vi "KB- 颜色分类.vi"(10 "Fitted Circle (Inner Find Circular Edge 2)":T3, 11 "image in":T1(plugin-control)) -> (2 "输出簇":cluster{"金色个数":i32, "银色个数":i32, "黑色个数":i32}, 3 "image in 2":T1(plugin-control))   [LabVIEW 2015]
uses:
  <vilib>/vision/NI_Vision_Development_Module.lvlib
panel:
  out "黑色":i32
  out "银色":i32
  out "金色个数":i32
  out "数组":T2(array[cluster])
  out "Image Pixels (U32)":u32[][](array[numeric])
  # "Overview: Demonstrates how to use the IMAQ Classify function with a color classifier file to classify the color within a Region of Interest (ROI).\nRequirements: Vision Development Software.\nInstructions:\n1. Run the VI.\n2. Draw a ROI in the image to see what class the color is associated with and the score. Hold down <Ctrl> to select more than one ROI."
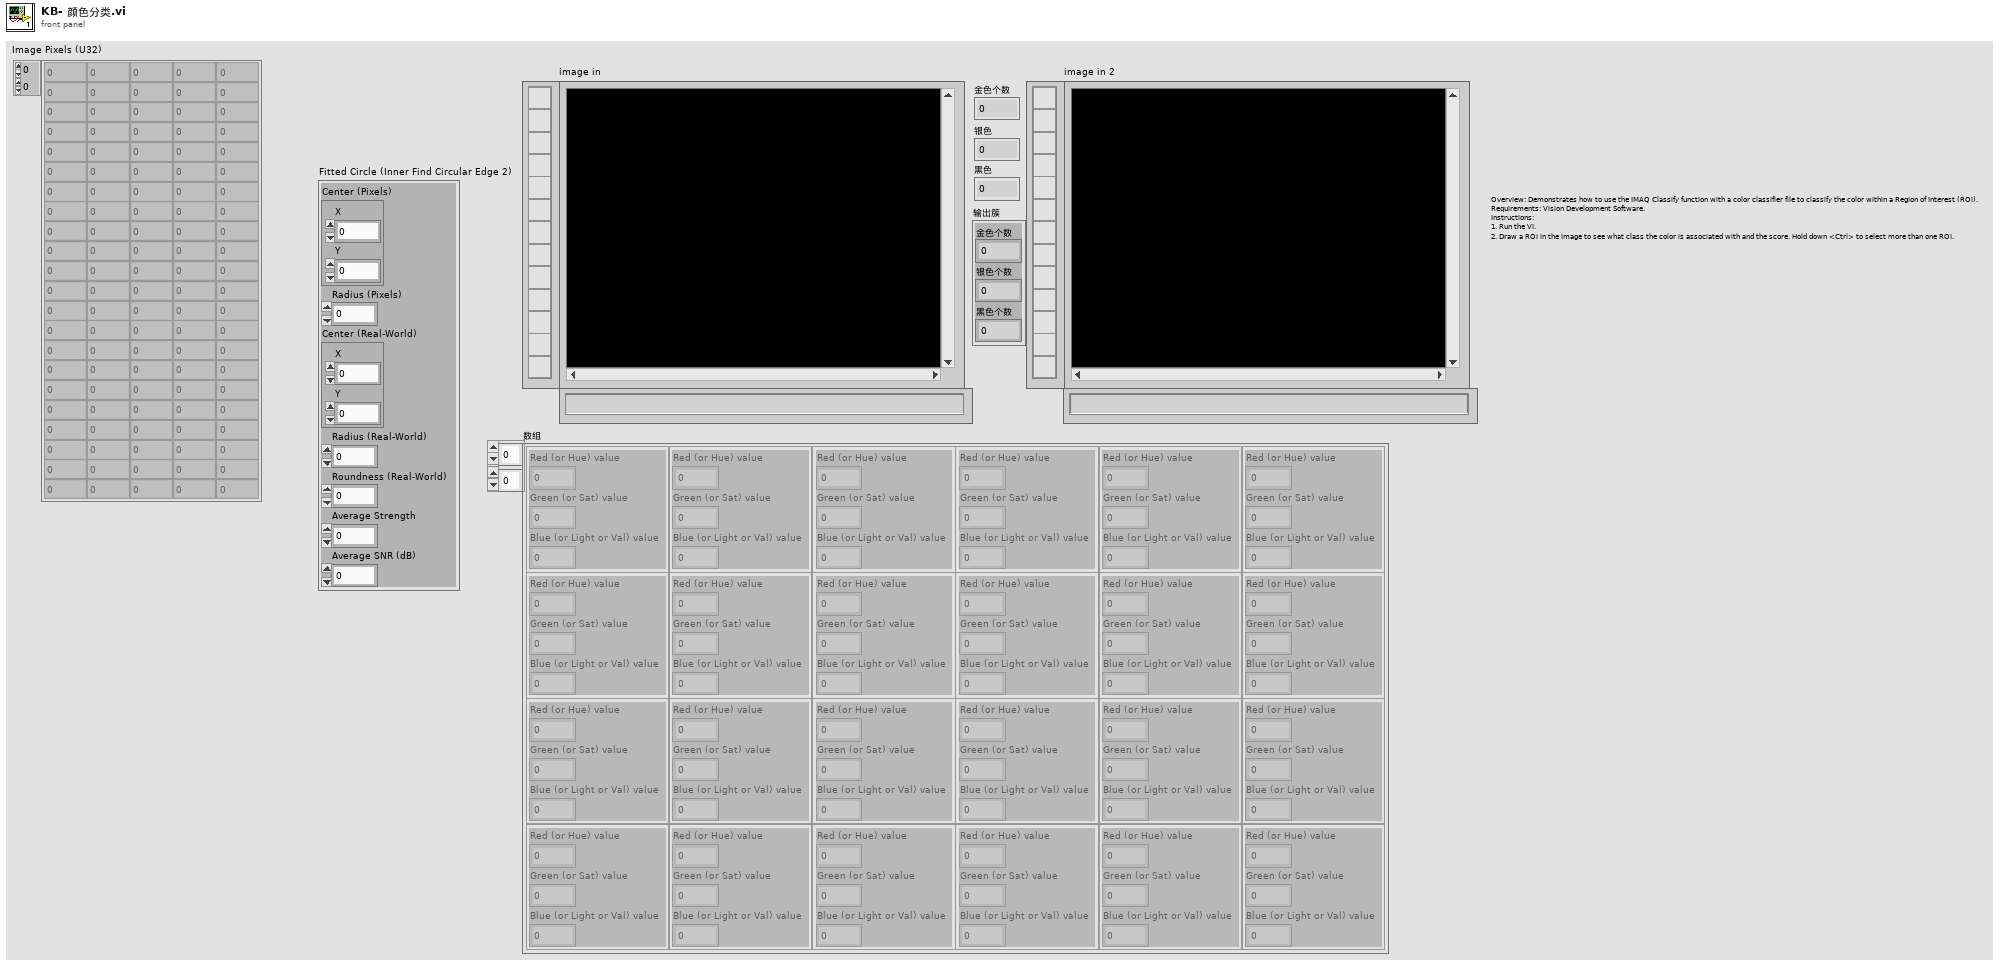
[diagram p1: front panel]
types:
  T1 = typedef "IMAQ Image.ctl" = refnum<image>
  T2 = cluster{"Red (or Hue) value":u8, "Green (or Sat) value":u8, "Blue (or Light or Val) value":u8}[][]
  T3 = cluster{"Center (Pixels)":cluster{"X":sgl, "Y":sgl}, "Radius (Pixels)":dbl, "Center (Real-World)":cluster{"X":sgl, "Y":sgl}, "Radius (Real-World)":dbl, "Roundness (Real-World)":dbl, "Average Strength":dbl, "Average SNR (dB)":dbl}
  T4 = typedef "Image Type" = u32
  T5 = cluster{"Red (or Hue) value":u8, "Green (or Sat) value":u8, "Blue (or Light or Val) value":u8}
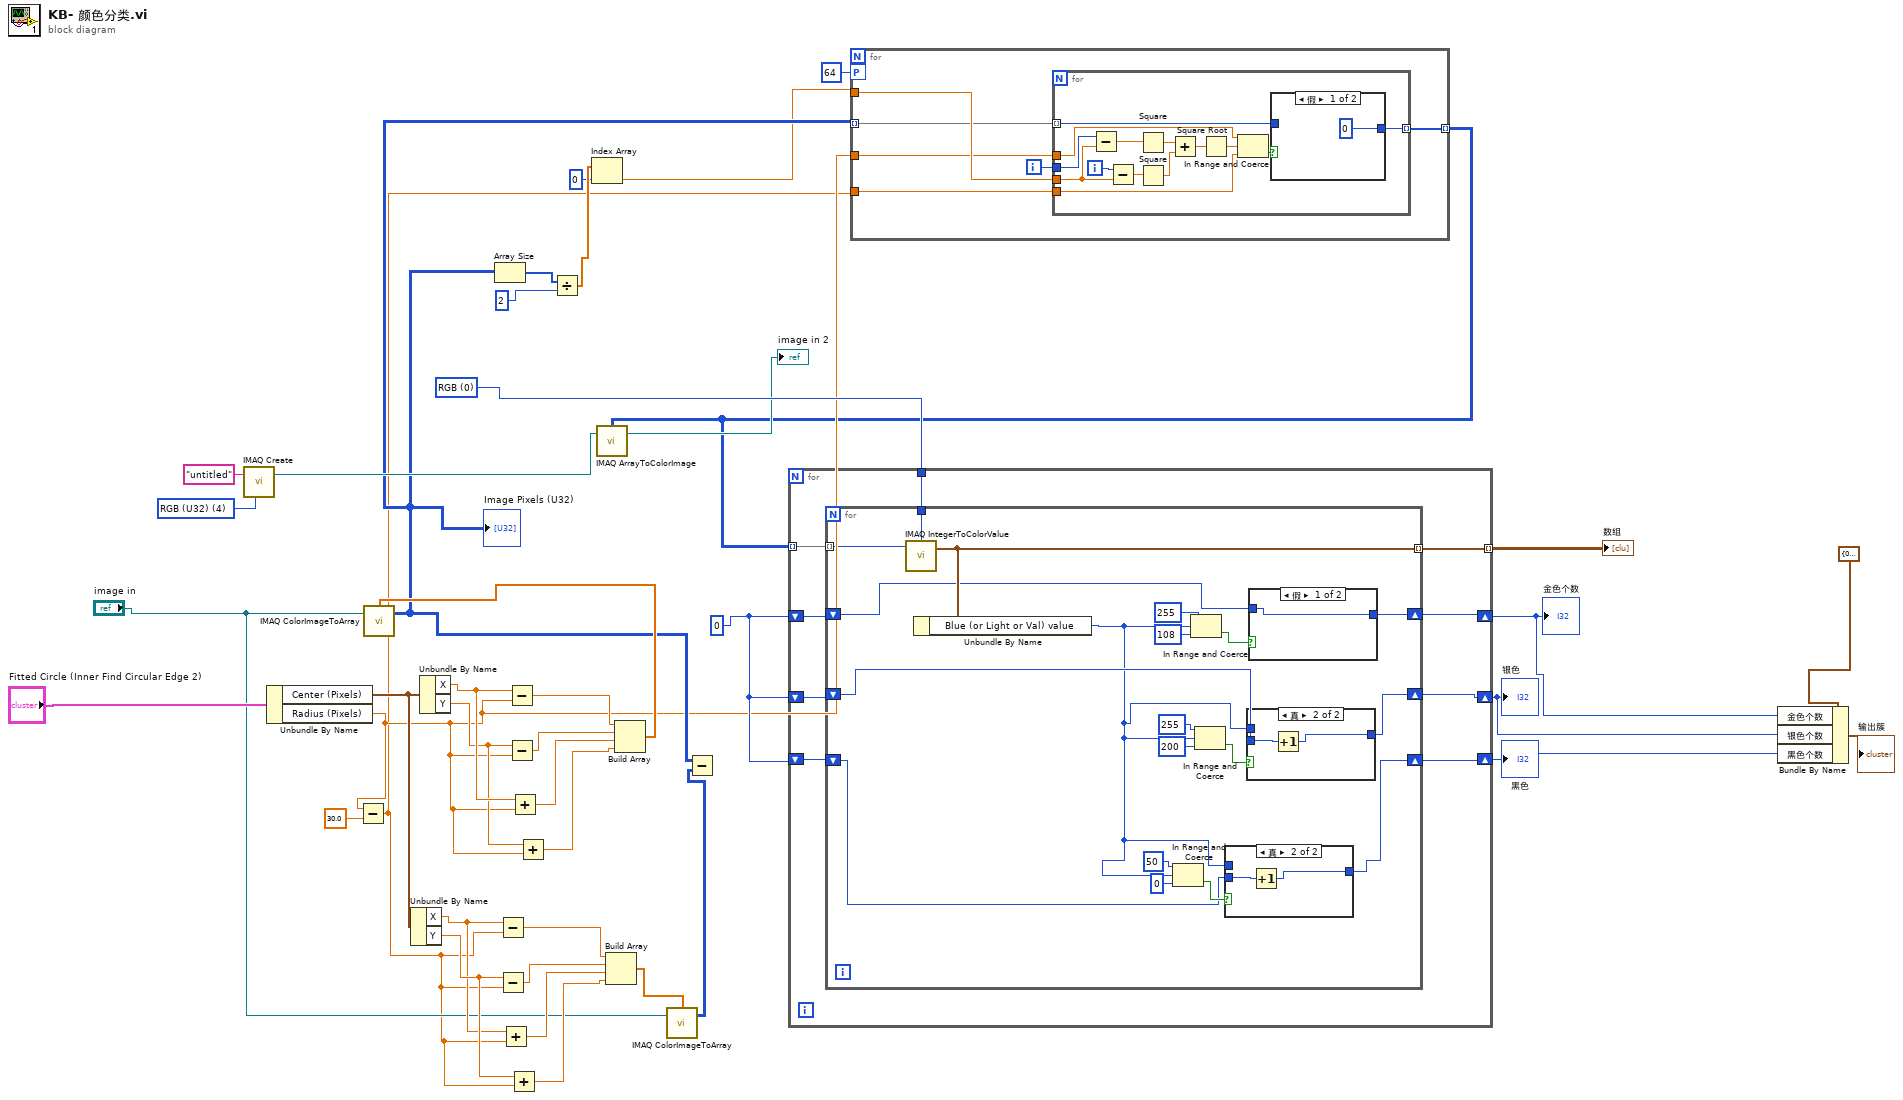
[diagram p0: block diagram]
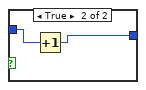
[diagram p4: hidden frame]
diagram:
  w18 = T4 4 items=["Grayscale (U8)", "Grayscale (I16)", "Grayscale (SGL)", "Complex (CSG)", "RGB (U32)", "HSL (U32)", "RGB (U64)", "Grayscale (U16)"] ("Image Type")
  w31 = 0
  w33 = u16 0 items=["RGB", "HSL", "HSV", "HSI"] ("Color Mode")
  n1 = call "IMAQ Create"("Image Name"="untitled", "Image Type"=w18) -> ("New Image"=w17:T1)  [unwired: 3 in, 1 out]
  n2 = Unbundle By Name("Fitted Circle (Inner Find Circular Edge 2)") -> ("Center (Pixels)"=w24:cluster{"X":sgl, "Y":sgl}, "Radius (Pixels)"=w9:dbl)
  n3 = Subtract(x=w9, y=30.0) -> (x-y=w8:dbl)
  n4 = Unbundle By Name(w24) -> ("X"=w25:sgl, "Y"=w26:sgl)
  n5 = Unbundle By Name(w24) -> ("X"=w40:sgl, "Y"=w39:sgl)
  n6 = Subtract(x=w25, y=w8) -> (x-y=w27:dbl)
  n7 = Subtract(x=w26, y=w8) -> (x-y=w28:dbl)
  n8 = Add(x=w25, y=w8) -> (x+y=w29:dbl)
  n9 = Subtract(x=w40, y=w9) -> (x-y=w38:dbl)
  n10 = Subtract(x=w39, y=w9) -> (x-y=w37:dbl)
  n11 = Add(x=w26, y=w8) -> (x+y=w30:dbl)
  n12 = Add(x=w40, y=w9) -> (x+y=w36:dbl)
  n13 = Add(x=w39, y=w9) -> (x+y=w35:dbl)
  n14 = Build Array(w27, w28, w29, w30) -> (w22:dbl[])
  n15 = Build Array(w38, w37, w36, w35) -> (w34:dbl[])
  n16 = call "IMAQ ColorImageToArray"("Optional Rectangle"=w34, "Image"="image in") -> ("Image Pixels (U32)"=w13:u32[][])  [unwired: 2 in, 2 out]
  "Image Pixels (U32)" <- w13
  n17 = Array Size(array=w13) -> (size(s)=w15:i32[])
  n18 = Divide(x=w15, y=2) -> (x/y=w12:dbl[])
  n19 = Index Array(array=w12, index=0 ("索引")) -> (element=w10:dbl)
  n20 = call "IMAQ ColorImageToArray"("Optional Rectangle"=w22, "Image"="image in") -> ("Image Pixels (U32)"=w20:u32[][])  [unwired: 2 in, 2 out]
  n21 = Subtract(x=w13, y=w20) -> ()  [unwired: 1 out]
  n22 = for {
    tunnel: w13 -> [w43] mode=indexing
    tunnel: w8 -> [w44]
    tunnel: w10 -> [w46]
    tunnel: w9 -> [w45]
    tunnel: [w42] -> w6 mode=indexing
    workers-P: 64 -> [_]
    i -> [w47]
    n23 = for {
      tunnel: w47 -> [w61]
      tunnel: w46 -> [w58]
      tunnel: w45 -> [w52]
      tunnel: w44 -> [w51]
      tunnel: w43 -> [w49] mode=indexing
      tunnel: [w48] -> w42 mode=indexing
      i -> [w59]
      n24 = Subtract(x=w61, y=w58) -> (x-y=w60:dbl)
      n25 = Subtract(x=w59, y=w58) -> (x-y=w57:dbl)
      n26 = Square(x=w60) -> (x^2=w55:dbl)
      n27 = Square(x=w57) -> (x^2=w56:dbl)
      n28 = Add(x=w55, y=w56) -> (x+y=w54:dbl)
      n29 = Square Root(x=w54) -> (sqrt(x)=w53:dbl)
      n30 = In Range and Coerce(upper limit=w52, x=w53, lower limit=w51) -> (In Range?=w50:bool)  [unwired: 1 out]
      n31 = case shown="假" w50 {
        tunnel: w49 -> [_ w63]
        tunnel: [u32 0 w63] -> w48
        frame False {
        }
        frame True {
        }
      }
    }
  }
  n32 = call "IMAQ ArrayToColorImage"("Image Pixels (U32)"=w6, "Image"=w17) -> ("Image Out"=→"image in 2":T1)  [unwired: 3 in, 1 out]
  n33 = for {
    tunnel: w6 -> [w72] mode=indexing
    tunnel: w33 -> [w71]
    tunnel: [w70] -> w32 mode=indexing
    shift-right: [w68] -> w4
    shift-left: w31 -> [w69]
    shift-right: [w64] -> w3
    shift-left: w31 -> [w67]
    shift-right: [w65] -> w2
    shift-left: w31 -> [w66]
    n34 = for {
      tunnel: w72 -> [w91] mode=indexing
      tunnel: w71 -> [w90]
      tunnel: [w89] -> w70 mode=indexing
      shift-right: [w84] -> w68
      shift-left: w69 -> [w85]
      shift-right: [w80] -> w64
      shift-left: w67 -> [w79]
      shift-right: [w75] -> w65
      shift-left: w66 -> [w73]
      n35 = call "IMAQ IntegerToColorValue"("U32 value"=w91, "Color Mode"=w90) -> ("Color Value"=w89:T5)  [unwired: 3 in, 3 out]
      n36 = Unbundle By Name(w89) -> ("Blue (or Light or Val) value"=w76:u8)
      n37 = In Range and Coerce(upper limit=u8 50 ("上限"), x=w76, lower limit=u8 0 ("下限")) -> (In Range?=w74:bool)  [unwired: 1 out]
      n38 = In Range and Coerce(upper limit=u8 255 ("上限"), x=w76, lower limit=u8 108 ("下限")) -> (In Range?=w86:bool)  [unwired: 1 out]
      n39 = In Range and Coerce(upper limit=u8 255 ("上限"), x=w76, lower limit=u8 200 ("下限")) -> (In Range?=w81:bool)  [unwired: 1 out]
      n40 = case shown="真" w74 {
        tunnel: w76 -> [_ _]
        tunnel: [w92 w94] -> w75
        tunnel: w73 -> [w92 w93]
        frame False {
        }
        frame True {
          n41 = Increment(x=w93) -> (x+1=w94:i32)
        }
      }
      n42 = case shown="真" w81 {
        tunnel: w76 -> [_ _]
        tunnel: [w95 w97] -> w80
        tunnel: w79 -> [w95 w96]
        frame False {
        }
        frame True {
          n43 = Increment(x=w96) -> (x+1=w97:i32)
        }
      }
      n44 = case shown="假" w86 {
        tunnel: w85 -> [w98 w100]
        tunnel: [w98 w99] -> w84
        frame False {
        }
        frame True {
          n45 = Increment(x=w100) -> (x+1=w99:i32)
        }
      }
    }
  }
  "数组" <- w32
  "金色个数" <- w4
  "银色" <- w3
  "黑色" <- w2
  n46 = Bundle By Name(cluster=cluster{"金色个数":i32, "银色个数":i32, "黑色个数":i32} {"金色个数"=0, "银色个数"=0, "黑色个数"=0}, "金色个数"=w4, "银色个数"=w3, "黑色个数"=w2) -> (→"输出簇":cluster{"金色个数":i32, "银色个数":i32, "黑色个数":i32})
